vi "ColorGraphScale.vi"(11 "GraphRef":refnum<vi>) -> ()   [LabVIEW 2019]
uses:
  <vilib>/Utility/config.llb/Write Key (String).vi
  <vilib>/Utility/config.llb/Read Key (String).vi
  <vilib>/Utility/config.llb/NI_LVConfig.lvlib
panel:
  in  "Available Scales":u16(ring)
  in  "Load":bool
  in  "Scale Name":string
  in  "Save":bool
  in  "Add Aft":bool
  in  "SetMarker":bool
  in  "Rem":bool
  in  "Add Bef":bool
  in  "Max":dbl
  in  "Min":dbl
  in  "Marker Index":u16(ring) items=["1", "2", "3", "4", "5"]
  in  "TestData":dbl[][](array[numeric])
  in  "Test Data":bool
  in  "Quit":bool
  in  "InitProg":bool
  in  "Color":u32(colorbox)
  in  "ColorVal":u32 caption="Color Value"
  in  "MarkVal":dbl caption="Marker Value"
  out "error out":errorcluster caption="sortie d'erreur"
  in  "error in (no error)":errorcluster
  in  "Z.MarkVal":cluster{"MarkerVal":dbl, "ColorVal":u32}[](array[cluster])
  out "Graphe d'intensité":dbl[][](graph)
  # "ColorScale"
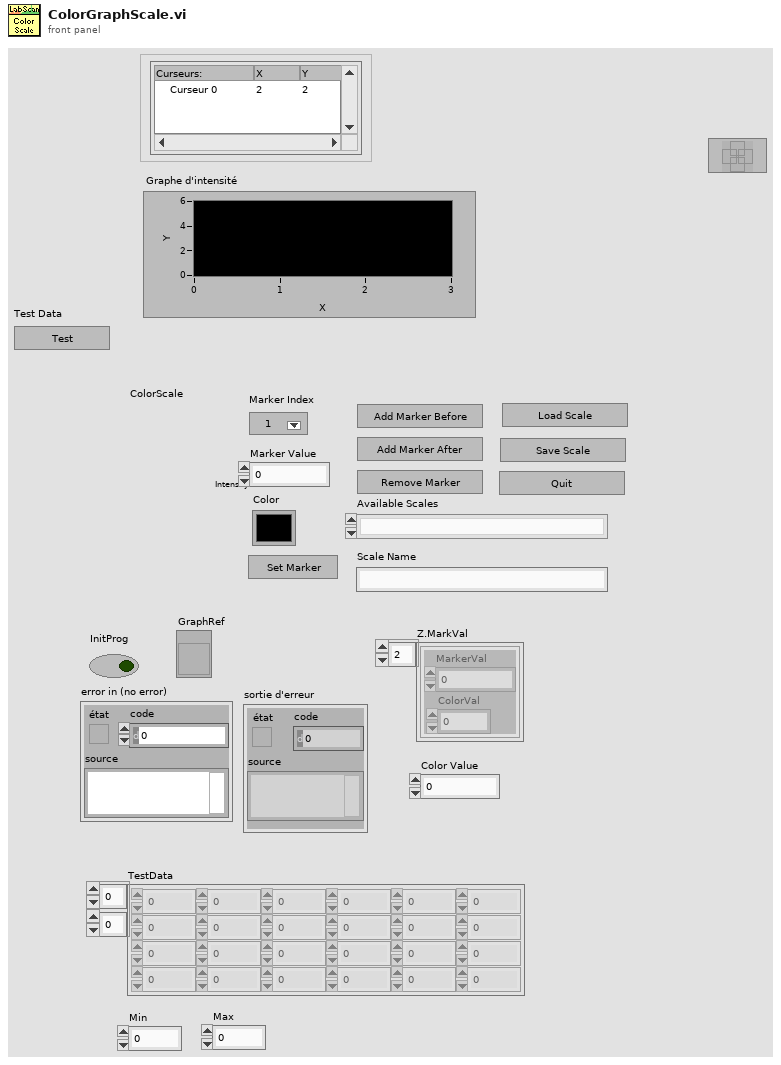
[diagram p1: front panel]
types:
  T1 = enum16{"Répertoire du VI actuel", "Répertoire du parent 1", "Répertoire du parent 2", "Répertoire du parent 3"}
  T2 = typedef "NI_LVConfig.lvlib/Config Data RefNum.ctl" = refnum<k1>
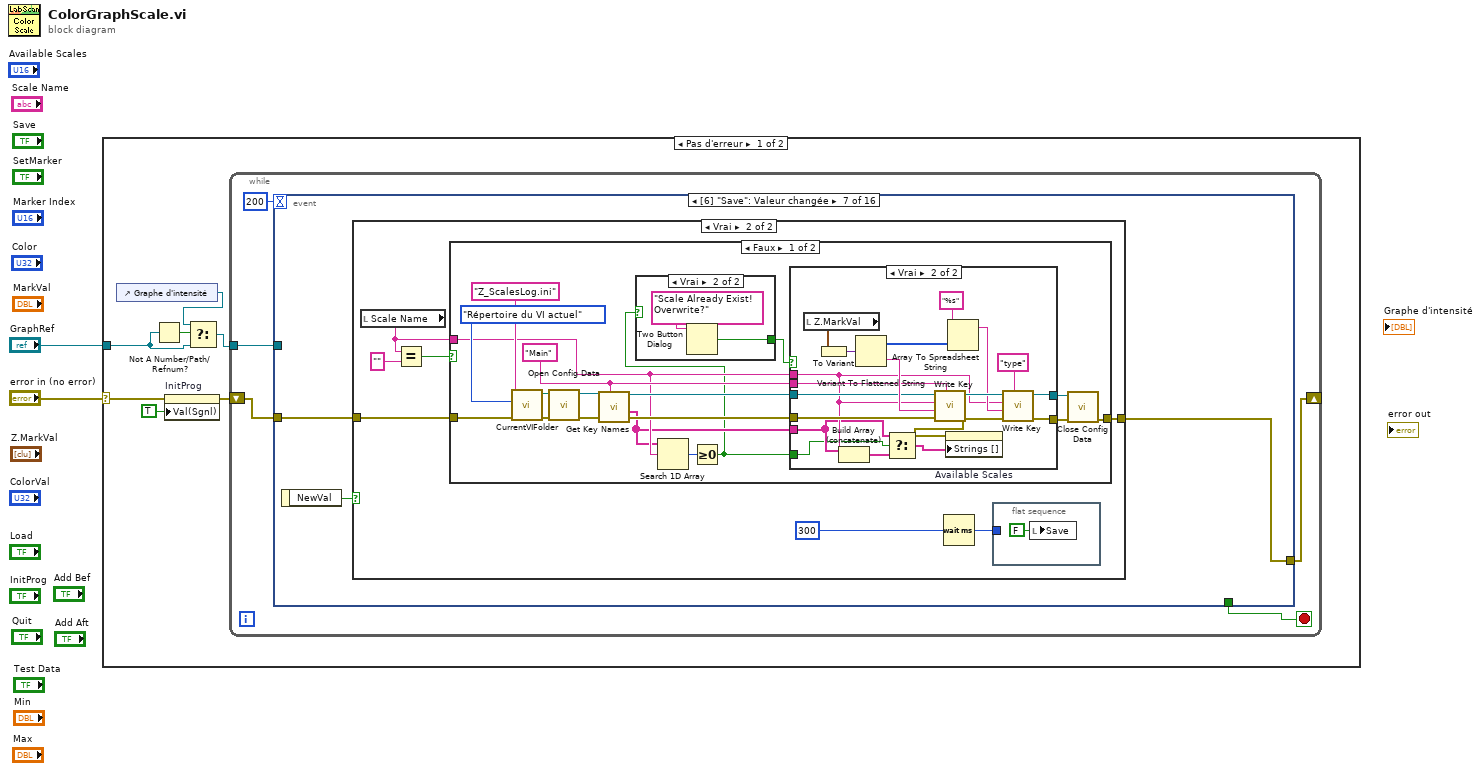
[diagram p0: block diagram]
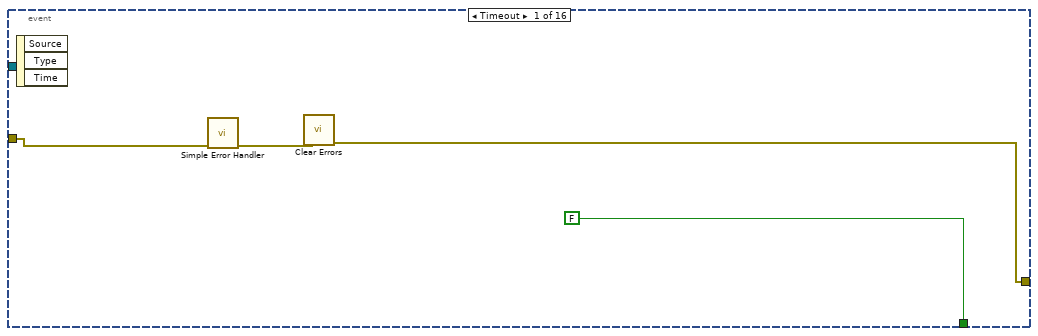
[diagram p2: hidden frame]
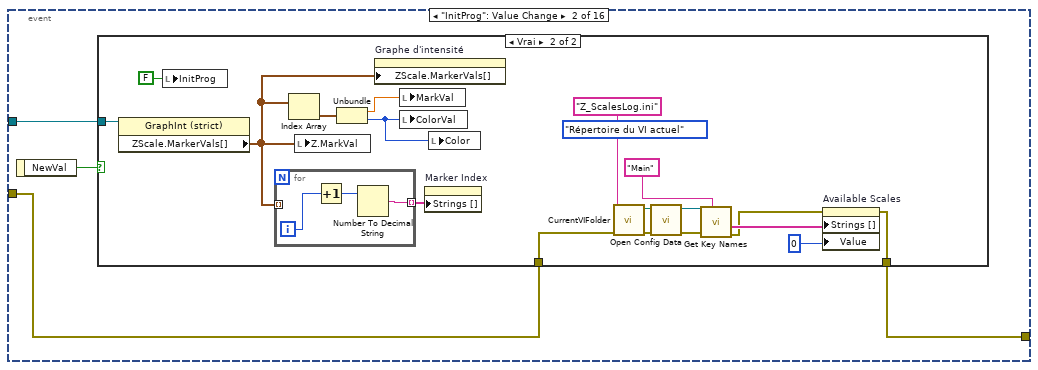
[diagram p3: hidden frame]
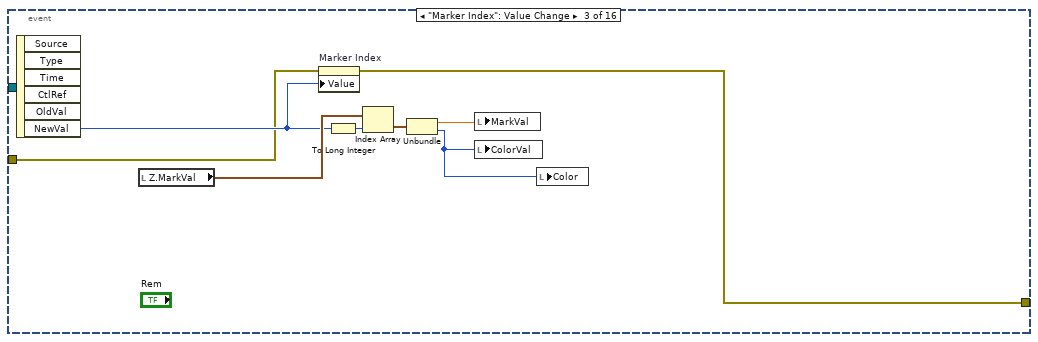
[diagram p5: hidden frame]
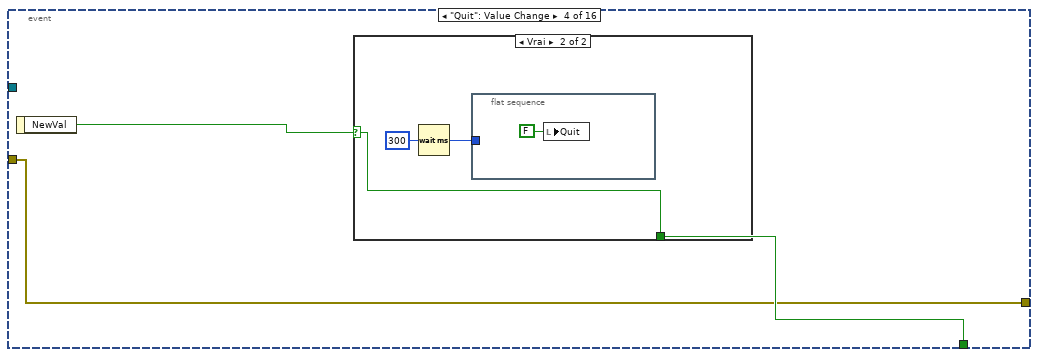
[diagram p6: hidden frame]
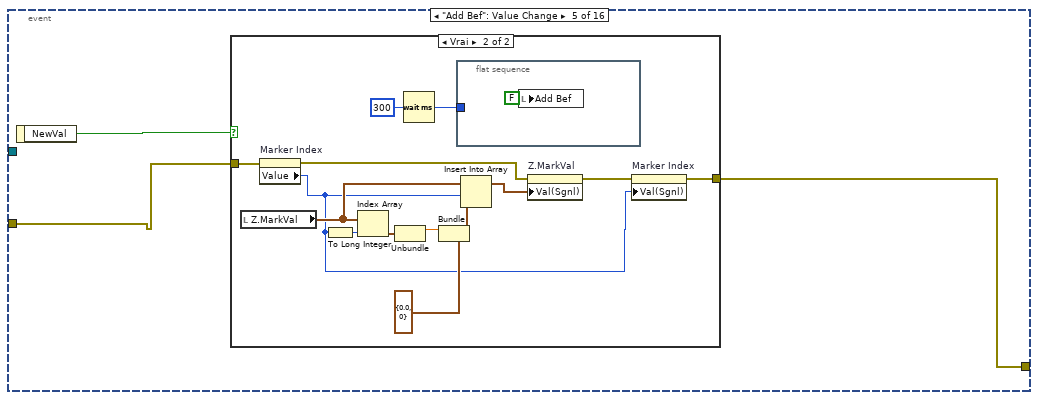
[diagram p8: hidden frame]
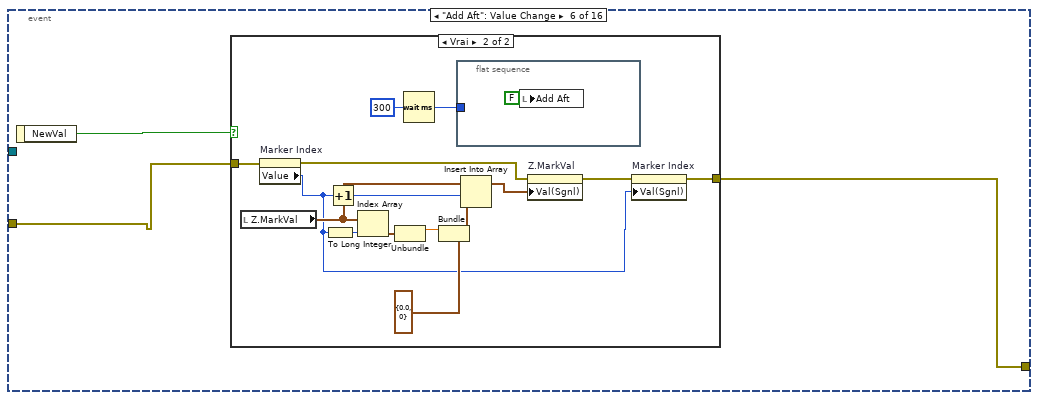
[diagram p10: hidden frame]
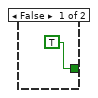
[diagram p13: hidden frame]
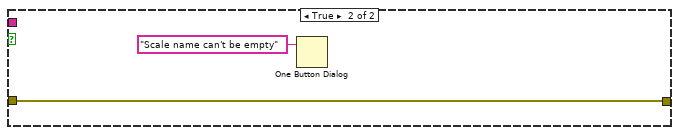
[diagram p15: hidden frame]
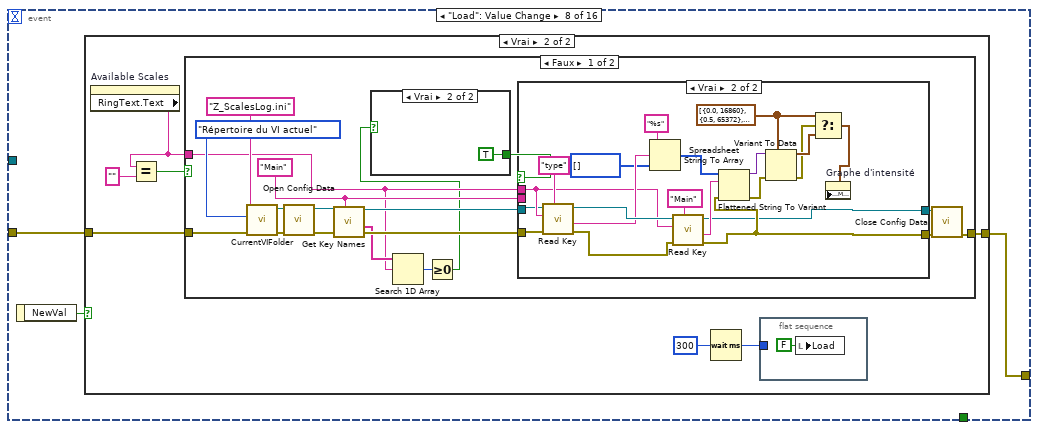
[diagram p16: hidden frame]
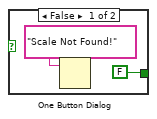
[diagram p18: hidden frame]
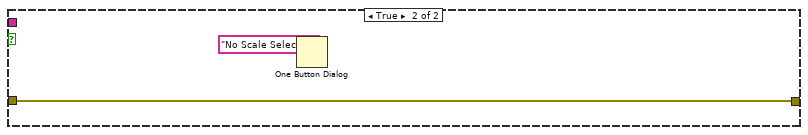
[diagram p20: hidden frame]
diagram:
  n1 = case shown="Pas d'erreur" "error in (no error)" {
    selector: "error in (no error)" -> [w9 _]
    tunnel: "GraphRef" -> [w5 _]
    frame No Error {
      n2 = control-ref of="Graphe d'intensité"() -> (w4:refnum<vi>)
      n3 = Not A Number/Path/Refnum?(number/path/refnum=w5) -> (NaN/Path/Refnum?=w6:bool)
      n4 = property on="InitProg" class="Bool (strict)"(error in=w9, "Val(Sgnl)"=TRUE ("Valeur (Signalisation)")) -> (error out=w8:errorcluster)  [unwired: 1 in, 1 out]
      n5 = Select(t=w4, s=w6, f=w5) -> (s? t:f=w3:refnum<vi>)
      n6 = while {
        shift-right: [w12] -> _
        shift-left: w8 -> [w11]
        tunnel: w3 -> [w10]
        stop <- w13 stop-if-true
        n7 = event shown="[6] \"Save\": Valeur changée" {
          selector: _ -> [_ _ _ _ _ _ _ _ _ _ _ _ _ _ _ _]
          dyn-events: _ -> [_ _ _ _ _ _ _ _ _ _ _ _ _ _ _ _]
          timeout: 200 -> [_ _ _ _ _ _ _ _ _ _ _ _ _ _ _ _]
          tunnel: [FALSE _ _ w54 _ _ _ _ _ _ _ _ _ _ _ _] -> w13
          tunnel: [w15 w20 w45 w53 w62 w81 w101 w157 w213 _ _ _ w243 w264 _ _] -> w12
          tunnel: w11 -> [w17 w19 w46 w53 w61 w80 w100 w156 w214 _ _ _ w247 w259 _ _]
          tunnel: w10 -> [_ w21 _ _ _ _ _ _ _ _ _ _ _ w263 _ _]
          event Timeout {
            n8 = event-data() -> ()  [unwired: 1 in, 3 out]
            n9 = call <vilib>:"Simple Error Handler.vi"("error in (no error)"=w17) -> ("error out"=w16:errorcluster)  [unwired: 4 in, 4 out]
            n10 = call <vilib>:"Clear Errors.vi"("error in (no error)"=w16) -> ("error out"=w15:errorcluster)  [unwired: 5 in, 1 out]
          }
          event "InitProg": Value Change {
            n11 = event-data() -> ("NewVal"=w22:bool)  [unwired: 1 in]
            n12 = case shown="Vrai" w22 {
              tunnel: w21 -> [_ w40]
              tunnel: w19 -> [w23 w26]
              tunnel: [w23 w25] -> w20
              frame False {
              }
              frame True {
                (unwired) T1."Répertoire du VI actuel" ("Source")
                n13 = property class="GraphInt (strict)"(reference=w40) -> ("ZScale.MarkerVals[]"=w35:cluster{dbl, u32}[])  [unwired: 1 in, 2 out]
                n14 = local write "InitProg"(FALSE ("InitProg")) -> ()
                n15 = for {
                  tunnel: [w43] -> w36 mode=indexing
                  tunnel: w35 -> [_] mode=indexing
                  i -> [w44]
                  n16 = Increment(x=w44) -> (x+1=w42:i32)
                  n17 = Number To Decimal String(number=w42) -> (decimal integer string=w43:string)  [unwired: 1 in]
                }
                n18 = Index Array(array=w35) -> (element=w39:cluster{dbl, u32})  [unwired: 1 in]
                n19 = local write "Z.MarkVal"(w35) -> ()
                n20 = Unbundle(w39) -> (w37:dbl, w38:u32)
                n21 = property on="Graphe d'intensité" class="GraphInt (strict)"("ZScale.MarkerVals[]"=w35) -> ()  [unwired: 2 in, 2 out]
                n22 = local write "MarkVal"(w37) -> ()
                n23 = local write "ColorVal"(w38) -> ()
                n24 = property on="Marker Index" class="MDér (strict)"("Strings []"=w36) -> ()  [unwired: 2 in, 2 out]
                n25 = local write "Color"(w38) -> ()
                n26 = call <userlib>:"CurrentVIFolder.vi"("error in (no error)"=w26, "NomFichier"="Z_ScalesLog.ini") -> ("error out"=w32:errorcluster, "Chemin"=w33:path)  [unwired: 7 in, 1 out]
                n27 = call <vilib>:"Open Config Data.vi"("error in (no error)"=w32, "configuration file path"=w33) -> ("error out"=w31:errorcluster, "refnum"=w30:T2)  [unwired: 7 in, 1 out]
                n28 = call <vilib>:"Get Key Names.vi"("section"="Main", "error in (no error)"=w31, "refnum"=w30) -> ("error out"=w27:errorcluster, "key names"=w28:string[])  [unwired: 5 in, 2 out]
                n29 = property on="Available Scales" class="MDér (strict)"(error in=w27, "Strings []"=w28, "Value"=0) -> (error out=w25:errorcluster)  [unwired: 1 in, 1 out]
              }
            }
          }
          event "Marker Index": Value Change {
            n30 = event-data() -> ("NewVal"=w47:u16)  [unwired: 1 in, 5 out]
            n31 = local read "Z.MarkVal"() -> (w52:cluster{"MarkerVal":dbl, "ColorVal":u32}[])
            n32 = property on="Marker Index" class="MDér (strict)"(error in=w46, "Value"=w47) -> (error out=w45:errorcluster)  [unwired: 1 in, 1 out]
            n33 = To Long Integer(number=w47) -> (32bit integer=w51:i32)
            n34 = Index Array(array=w52, index=w51) -> (element=w50:cluster{"MarkerVal":dbl, "ColorVal":u32})
            n35 = Unbundle(w50) -> ("MarkerVal"=w49:dbl, "ColorVal"=w48:u32)
            n36 = local write "MarkVal"(w49) -> ()
            n37 = local write "ColorVal"(w48) -> ()
            n38 = local write "Color"(w48) -> ()
          }
          event "Quit": Value Change {
            n39 = event-data() -> ("NewVal"=w55:bool)  [unwired: 1 in]
            n40 = case shown="Vrai" w55 {
              selector: w55 -> [w56 w59]
              tunnel: [w56 w59] -> w54
              frame False {
              }
              frame True {
                n41 = Wait (ms)(milliseconds to wait=u32 300 ("attente (ms)")) -> (millisecond timer value=w57:u32)
                n42 = flat-sequence {
                  tunnel: w57 -> [_]
                  frame #0 {
                    n43 = local write "Quit"(FALSE ("Quit")) -> ()
                  }
                }
              }
            }
          }
          event "Add Bef": Value Change {
            n44 = event-data() -> ("NewVal"=w63:bool)  [unwired: 1 in]
            n45 = case shown="Vrai" w63 {
              tunnel: w61 -> [w64 w73]
              tunnel: [w64 w74] -> w62
              frame False {
              }
              frame True {
                n46 = local read "Z.MarkVal"() -> (w70:cluster{"MarkerVal":dbl, "ColorVal":u32}[])
                n47 = property on="Marker Index" class="MDér (strict)"(error in=w73) -> (error out=w72:errorcluster, "Value"=w66:u16)  [unwired: 1 in, 1 out]
                n48 = To Long Integer(number=w66) -> (32bit integer=w65:i32)
                n49 = Index Array(array=w70, index=w65) -> (element=w69:cluster{"MarkerVal":dbl, "ColorVal":u32})
                n50 = Unbundle(w69) -> ("MarkerVal"=w67:dbl)  [unwired: 1 out]
                n51 = Wait (ms)(milliseconds to wait=u32 300 ("attente (ms)")) -> (millisecond timer value=w77:u32)
                n52 = Bundle(cluster=cluster{"MarkerVal":dbl, "ColorVal":u32} {"MarkerVal"=0.0, "ColorVal"=0}, "MarkerVal"=w67) -> (w68:cluster{"MarkerVal":dbl, "ColorVal":u32})  [unwired: 1 in]
                n53 = flat-sequence {
                  tunnel: w77 -> [_]
                  frame #0 {
                    n54 = local write "Add Bef"(FALSE ("Quit")) -> ()
                  }
                }
                n55 = Insert Into Array(array=w70, index=w66, new element=w68) -> (w75:cluster{"MarkerVal":dbl, "ColorVal":u32}[])
                n56 = property on="Z.MarkVal" class="Tabl (strict)"(error in=w72, "Val(Sgnl)"=w75) -> (error out=w76:errorcluster)  [unwired: 1 in, 1 out]
                n57 = property on="Marker Index" class="MDér (strict)"(error in=w76, "Val(Sgnl)"=w66) -> (error out=w74:errorcluster)  [unwired: 1 in, 1 out]
              }
            }
          }
          event "Add Aft": Value Change {
            n58 = event-data() -> ("NewVal"=w82:bool)  [unwired: 1 in]
            n59 = case shown="Vrai" w82 {
              tunnel: w80 -> [w83 w93]
              tunnel: [w83 w94] -> w81
              frame False {
              }
              frame True {
                n60 = local read "Z.MarkVal"() -> (w90:cluster{"MarkerVal":dbl, "ColorVal":u32}[])
                n61 = property on="Marker Index" class="MDér (strict)"(error in=w93) -> (error out=w92:errorcluster, "Value"=w84:u16)  [unwired: 1 in, 1 out]
                n62 = To Long Integer(number=w84) -> (32bit integer=w86:i32)
                n63 = Increment(x=w84) -> (x+1=w85:u16)
                n64 = Index Array(array=w90, index=w86) -> (element=w89:cluster{"MarkerVal":dbl, "ColorVal":u32})
                n65 = Unbundle(w89) -> ("MarkerVal"=w87:dbl)  [unwired: 1 out]
                n66 = Wait (ms)(milliseconds to wait=u32 300 ("attente (ms)")) -> (millisecond timer value=w97:u32)
                n67 = Bundle(cluster=cluster{"MarkerVal":dbl, "ColorVal":u32} {"MarkerVal"=0.0, "ColorVal"=0}, "MarkerVal"=w87) -> (w88:cluster{"MarkerVal":dbl, "ColorVal":u32})  [unwired: 1 in]
                n68 = flat-sequence {
                  tunnel: w97 -> [_]
                  frame #0 {
                    n69 = local write "Add Aft"(FALSE ("Quit")) -> ()
                  }
                }
                n70 = Insert Into Array(array=w90, index=w85, new element=w88) -> (w95:cluster{"MarkerVal":dbl, "ColorVal":u32}[])
                n71 = property on="Z.MarkVal" class="Tabl (strict)"(error in=w92, "Val(Sgnl)"=w95) -> (error out=w96:errorcluster)  [unwired: 1 in, 1 out]
                n72 = property on="Marker Index" class="MDér (strict)"(error in=w96, "Val(Sgnl)"=w84) -> (error out=w94:errorcluster)  [unwired: 1 in, 1 out]
              }
            }
          }
          event "Save": Value Change {
            n73 = event-data() -> ("NewVal"=w102:bool)  [unwired: 1 in]
            n74 = case shown="Vrai" w102 {
              tunnel: [w103 w109] -> w101
              tunnel: w100 -> [w103 w110]
              frame False {
              }
              frame True {
                n75 = local read "Scale Name"() -> (w104:string)
                n76 = Equal?(x=w104, y="") -> (x = y?=w105:bool)
                n77 = case shown="Faux" w105 {
                  tunnel: w110 -> [w126 w153]
                  tunnel: [w114 w153] -> w109
                  tunnel: w104 -> [w118 _]
                  frame False {
                    w119 = "Main" ("section")
                    n78 = call <userlib>:"CurrentVIFolder.vi"("error in (no error)"=w126, "Source"=T1."Répertoire du VI actuel", "NomFichier"="Z_ScalesLog.ini") -> ("error out"=w124:errorcluster, "Chemin"=w125:path)  [unwired: 6 in, 1 out]
                    n79 = call <vilib>:"Open Config Data.vi"("error in (no error)"=w124, "configuration file path"=w125) -> ("error out"=w123:errorcluster, "refnum"=w122:T2)  [unwired: 7 in, 1 out]
                    n80 = call <vilib>:"Get Key Names.vi"("section"=w119, "error in (no error)"=w123, "refnum"=w122) -> ("error out"=w121:errorcluster, "key names"=w112:string[], "refnum out"=w120:T2)  [unwired: 5 in, 1 out]
                    n81 = Search 1D Array(1D array=w112, element=w118) -> (index of element=w117:i32)  [unwired: 1 in]
                    n82 = Greater Or Equal To 0?(x=w117) -> (x >= 0?=w111:bool)
                    n83 = case shown="Vrai" w111 {
                      tunnel: [TRUE ("T button?") w130] -> w113
                      frame False {
                      }
                      frame True {
                        n84 = Two Button Dialog(message="Scale Already Exist! Overwrite?") -> (T button?=w130:bool)  [unwired: 2 in]
                      }
                    }
                    n85 = case shown="Vrai" w113 {
                      tunnel: w121 -> [w132 w144]
                      tunnel: w120 -> [w133 w143]
                      tunnel: w119 -> [_ w142]
                      tunnel: w118 -> [_ w138]
                      tunnel: [w132 w141] -> w116
                      tunnel: [w133 w140] -> w115
                      tunnel: w112 -> [_ w136]
                      tunnel: w111 -> [_ w135]
                      frame False {
                      }
                      frame True {
                        n86 = local read "Z.MarkVal"() -> (w152:cluster{"MarkerVal":dbl, "ColorVal":u32}[])
                        n87 = To Variant(anything=w152) -> (Variant=w151:variant)
                        n88 = Build Array (concatenate)(w136, w138) -> (w137:string[])
                        n89 = Variant To Flattened String(Variant=w151) -> (data string=w150:string, 1:w147:i16[])
                        n90 = Select(t=w136, s=w135, f=w137) -> (s? t:f=w134:string[])
                        n91 = call-poly <vilib>:"Write Key.vi"("section"=w142, "error in (no error)"=w144, "value"=w150, "key"=w138, "refnum"=w143) -> ("error out"=w139:errorcluster, "refnum out"=w148:T2)  [unwired: 4 in, 1 out]
                        n92 = property on="Available Scales" class="MDér (strict)"(error in=w139, "Strings []"=w134) -> ()  [unwired: 1 in, 2 out]
                        n93 = Array To Spreadsheet String(array=w147, 3:"%s" ("chaîne de format")) -> (spreadsheet string=w146:string)  [unwired: 1 in]
                        n94 = call-poly <vilib>:"Write Key.vi"("section"="type", "error in (no error)"=w139, "value"=w146, "key"=w138, "refnum"=w148) -> ("error out"=w141:errorcluster, "refnum out"=w140:T2)  [unwired: 4 in, 1 out]
                      }
                    }
                    n95 = call <vilib>:"Close Config Data.vi"("error in (no error)"=w116, "refnum"=w115) -> ("error out"=w114:errorcluster)  [unwired: 8 in, 1 out]
                  }
                  frame True {
                    n96 = One Button Dialog(message="Scale name can't be empty") -> ()  [unwired: 1 in, 1 out]
                  }
                }
                n97 = Wait (ms)(milliseconds to wait=u32 300 ("attente (ms)")) -> (millisecond timer value=w108:u32)
                n98 = flat-sequence {
                  tunnel: w108 -> [_]
                  frame #0 {
                    n99 = local write "Save"(FALSE ("Save")) -> ()
                  }
                }
              }
            }
          }
          event "Load": Value Change {
            n100 = event-data() -> ("NewVal"=w158:bool)  [unwired: 1 in]
            n101 = case shown="Vrai" w158 {
              tunnel: [w159 w165] -> w157
              tunnel: w156 -> [w159 w166]
              frame False {
              }
              frame True {
                n102 = property on="Available Scales" class="MDér (strict)"() -> ("RingText.Text"=w160:string)  [unwired: 2 in, 2 out]
                n103 = Equal?(x=w160, y="") -> (x = y?=w161:bool)
                n104 = case shown="Faux" w161 {
                  tunnel: w166 -> [w182 w210]
                  tunnel: [w169 w210] -> w165
                  tunnel: w160 -> [w173 _]
                  frame False {
                    w174 = "Main" ("section")
                    n105 = call <userlib>:"CurrentVIFolder.vi"("error in (no error)"=w182, "Source"=T1."Répertoire du VI actuel", "NomFichier"="Z_ScalesLog.ini") -> ("error out"=w180:errorcluster, "Chemin"=w181:path)  [unwired: 6 in, 1 out]
                    n106 = call <vilib>:"Open Config Data.vi"("error in (no error)"=w180, "configuration file path"=w181) -> ("error out"=w179:errorcluster, "refnum"=w178:T2)  [unwired: 7 in, 1 out]
                    n107 = call <vilib>:"Get Key Names.vi"("section"=w174, "error in (no error)"=w179, "refnum"=w178) -> ("error out"=w177:errorcluster, "key names"=w175:string[], "refnum out"=w176:T2)  [unwired: 5 in, 1 out]
                    n108 = Search 1D Array(1D array=w175, element=w173) -> (index of element=w172:i32)  [unwired: 1 in]
                    n109 = Greater Or Equal To 0?(x=w172) -> (x >= 0?=w168:bool)
                    n110 = case shown="Vrai" w168 {
                      tunnel: [FALSE TRUE ("T button?")] -> w167
                      frame False {
                        n111 = One Button Dialog(message="Scale Not Found!") -> ()  [unwired: 1 in, 1 out]
                      }
                      frame True {
                      }
                    }
                    n112 = case shown="Vrai" w167 {
                      tunnel: w177 -> [w188 w195]
                      tunnel: w176 -> [w189 w190]
                      tunnel: w174 -> [_ _]
                      tunnel: w173 -> [_ w193]
                      tunnel: [w188 w194] -> w171
                      tunnel: [w189 w192] -> w170
                      frame False {
                      }
                      frame True {
                        w198 = cluster{"MarkerVal":dbl, "ColorVal":u32}[] [{"MarkerVal"=0.0, "ColorVal"=16860}, {"MarkerVal"=0.5, "ColorVal"=65372}, {"MarkerVal"=1.0, "ColorVal"=16776793}] ("Z.MarkVal")
                        n113 = call-poly <vilib>:"Read Key.vi"("section"="type", "error in (no error)"=w195, "key"=w193, "refnum"=w190) -> ("error out"=w204:errorcluster, "value"=w205:string, "refnum out"=w206:T2)  [unwired: 4 in, 1 out]
                        n114 = Spreadsheet String To Array(format string="%s" ("chaîne de format"), spreadsheet string=w205, array type (2D Dbl)=i16[] [] ("chaîne de type")) -> (array=w202:i16[])  [unwired: 1 in]
                        n115 = call-poly <vilib>:"Read Key.vi"("section"="Main", "error in (no error)"=w204, "key"=w193, "refnum"=w206) -> ("error out"=w194:errorcluster, "value"=w208:string, "refnum out"=w192:T2)  [unwired: 4 in, 1 out]
                        n116 = Flattened String To Variant(4:w194, 6:w208, 7:w202) -> (0:w200:errorcluster, 3:w201:variant)
                        n117 = Variant To Data(error in=w200, type=w198, Variant=w201) -> (data=w197:cluster{"MarkerVal":dbl, "ColorVal":u32}[], error out=w196:errorcluster)
                        n118 = Select(t=w198, s=w196, f=w197) -> (s? t:f=w191:cluster{"MarkerVal":dbl, "ColorVal":u32}[])
                        n119 = property on="Graphe d'intensité" class="GraphInt (strict)"("ZScale.MarkerVals[]"=w191) -> ()  [unwired: 2 in, 2 out]
                      }
                    }
                    n120 = call <vilib>:"Close Config Data.vi"("error in (no error)"=w171, "refnum"=w170) -> ("error out"=w169:errorcluster)  [unwired: 8 in, 1 out]
                  }
                  frame True {
                    n121 = One Button Dialog(message="No Scale Selected") -> ()  [unwired: 1 in, 1 out]
                  }
                }
                n122 = Wait (ms)(milliseconds to wait=u32 300 ("attente (ms)")) -> (millisecond timer value=w164:u32)
                n123 = flat-sequence {
                  tunnel: w164 -> [_]
                  frame #0 {
                    n124 = local write "Load"(FALSE ("Save")) -> ()
                  }
                }
              }
            }
          }
          event "Rem": Value Change {
            n125 = event-data() -> ("NewVal"=w215:bool)  [unwired: 1 in]
            n126 = case shown="Vrai" w215 {
              tunnel: w214 -> [w216 w225]
              tunnel: [w216 w224] -> w213
              frame False {
              }
              frame True {
                n127 = property on="Marker Index" class="MDér (strict)"() -> ("Value"=w218:u16)  [unwired: 2 in, 2 out]
                n128 = local read "Z.MarkVal"() -> (w223:cluster{"MarkerVal":dbl, "ColorVal":u32}[])
                n129 = Wait (ms)(milliseconds to wait=u32 300 ("attente (ms)")) -> (millisecond timer value=w227:u32)
                n130 = Greater Than 0?(x=w218) -> (x > 0?=w219:bool)
                n131 = Delete From Array(array=w223, length=1 ("longueur"), index=w218) -> (array with subset deleted=w222:cluster{"MarkerVal":dbl, "ColorVal":u32}[])  [unwired: 1 out]
                n132 = flat-sequence {
                  tunnel: w227 -> [_]
                  frame #0 {
                    n133 = local write "Rem"(FALSE ("Quit")) -> ()
                  }
                }
                n134 = Decrement(x=w218) -> (x-1=w220:u16)
                n135 = Select(t=w220, s=w219, f=w218) -> (s? t:f=w217:u16)
                n136 = property on="Z.MarkVal" class="Tabl (strict)"(error in=w225, "Val(Sgnl)"=w222) -> (error out=w226:errorcluster)  [unwired: 1 in, 1 out]
                n137 = property on="Marker Index" class="MDér (strict)"(error in=w226, "Val(Sgnl)"=w217) -> (error out=w224:errorcluster)  [unwired: 1 in, 1 out]
              }
            }
          }
          event "SetMarker": Value Change {
            n138 = event-data() -> ("NewVal"=w230:bool)  [unwired: 1 in, 5 out]
            n139 = case shown="Vrai" w230 {
              frame False {
              }
              frame True {
                n140 = local read "Z.MarkVal"() -> (w234:cluster{"MarkerVal":dbl, "ColorVal":u32}[])
                n141 = local read "Marker Index"() -> (w233:u16)
                n142 = local read "ColorVal"() -> (w235:u32)
                n143 = local read "MarkVal"() -> (w236:dbl)
                n144 = Wait (ms)(milliseconds to wait=u32 300 ("attente (ms)")) -> (millisecond timer value=w237:u32)
                n145 = flat-sequence {
                  tunnel: w237 -> [_]
                  frame #0 {
                    n146 = local write "SetMarker"(FALSE ("Quit")) -> ()
                  }
                }
                n147 = Bundle("MarkVal"=w236, "ColorVal"=w235) -> (w232:cluster{"MarkVal":dbl, "ColorVal":u32})  [unwired: 1 in]
                n148 = Replace Array Subset(array=w234, new element=w232, index=w233) -> (w231:cluster{"MarkerVal":dbl, "ColorVal":u32}[])
                n149 = property on="Z.MarkVal" class="Tabl (strict)"("Val(Sgnl)"=w231) -> ()  [unwired: 2 in, 2 out]
              }
            }
          }
          event "Color": Value Change {
            n150 = event-data() -> ("NewVal"=w240:u32)  [unwired: 1 in, 5 out]
            n151 = local write "ColorVal"(w240) -> ()
          }
          event "ColorVal": Value Change {
            n152 = event-data() -> ("NewVal"=w241:u32)  [unwired: 1 in, 5 out]
            n153 = local write "Color"(w241) -> ()
          }
          event "Test Data": Value Change {
            n154 = event-data() -> ("NewVal"=w250:bool)  [unwired: 1 in]
            n155 = case shown="Vrai" w250 {
              tunnel: [w251 w253] -> w248
              tunnel: w247 -> [w251 w253]
              tunnel: "TestData" -> [_ w252]
              frame False {
              }
              frame True {
                n156 = local write "Graphe d'intensité"(w252) -> ()
                n157 = Wait (ms)(milliseconds to wait=u32 300 ("attente (ms)")) -> (millisecond timer value=w255:u32)
                n158 = flat-sequence {
                  tunnel: w255 -> [_]
                  frame #0 {
                    n159 = local write "Test Data"(FALSE ("Quit")) -> ()
                  }
                }
              }
            }
            n160 = property on="Graphe d'intensité" class="GraphInt (strict)"(error in=w248) -> (error out=w244:errorcluster, "ZScale.MarkerVals[]"=w249:cluster{dbl, u32}[])  [unwired: 1 in, 1 out]
            n161 = property on="Z.MarkVal" class="Tabl (strict)"(error in=w244, "Val(Sgnl)"=w249) -> (error out=w246:errorcluster)  [unwired: 1 in, 1 out]
            n162 = property on="Marker Index" class="MDér (strict)"(error in=w246, "Val(Sgnl)"=u16 0 ("Valeur (Signalisation)")) -> (error out=w243:errorcluster)  [unwired: 1 in, 1 out]
          }
          event "Z.MarkVal": Value Change {
            n163 = event-data() -> ("NewVal"=w262:cluster{"MarkerVal":dbl, "ColorVal":u32}[])  [unwired: 1 in]
            n164 = property on="Marker Index" class="MDér (strict)"(error in=w259) -> (error out=w258:errorcluster, "Value"=w257:u16)  [unwired: 1 in, 1 out]
            n165 = for {
              tunnel: [w267] -> w265 mode=indexing
              tunnel: w262 -> [_] mode=indexing
              i -> [w268]
              n166 = Increment(x=w268) -> (x+1=w266:i32)
              n167 = Number To Decimal String(number=w266) -> (decimal integer string=w267:string)  [unwired: 1 in]
            }
            n168 = property on="Nœud de propriété" class="GraphInt (strict)"(reference=w263, error in=w258, "ZScale.MarkerVals[]"=w262) -> (error out=w261:errorcluster)  [unwired: 1 out]
            n169 = property on="Graphe d'intensité" class="GraphInt (strict)"(error in=w261, "ZScale.MarkerVals[]"=w262) -> (error out=w260:errorcluster)  [unwired: 1 in, 1 out]
            n170 = property on="Marker Index" class="MDér (strict)"(error in=w260, "Strings []"=w265, "Value"=w257) -> (error out=w264:errorcluster)  [unwired: 1 in, 1 out]
          }
          event "Min": Value Change {
            n171 = event-data() -> ("NewVal"=w278:dbl)  [unwired: 1 in]
            n172 = local read "Max"() -> (w279:dbl)
            n173 = local read "TestData"() -> (w280:dbl[][])
            n174 = Array Size(array=w280) -> (size(s)=w272:i32[])
            n175 = Subtract(x=w279, y=w278) -> (x-y=w277:dbl)
            n176 = Multiply Array Elements(1:w272) -> (0:w276:i32)
            n177 = Divide(x=w277, y=w276) -> (x/y=w275:dbl)
            n178 = for {
              N: w276 -> [_]
              tunnel: w275 -> [w282]
              tunnel: [w281] -> w274 mode=indexing
              i -> [w283]
              n179 = Multiply(x=w282, y=w283) -> (x*y=w281:dbl)
            }
            n180 = Index Array(array=w272) -> (element #1=w271:i32, element #2=w270:i32)  [unwired: 2 in]
            n181 = Reshape Array(w274, w271, w270) -> (w273:dbl[][])
            n182 = property on="Test Data" class="Bool (strict)"("Val(Sgnl)"=TRUE ("Valeur (Signalisation)")) -> ()  [unwired: 2 in, 2 out]
            n183 = local write "TestData"(w273) -> ()
          }
          event "Max": Value Change {
            n184 = event-data() -> ("NewVal"=w285:dbl)  [unwired: 1 in]
            n185 = local read "Min"() -> (w284:dbl)
            n186 = local read "TestData"() -> (w295:dbl[][])
            n187 = Array Size(array=w295) -> (size(s)=w289:i32[])
            n188 = Subtract(x=w285, y=w284) -> (x-y=w294:dbl)
            n189 = Multiply Array Elements(1:w289) -> (0:w293:i32)
            n190 = Divide(x=w294, y=w293) -> (x/y=w292:dbl)
            n191 = for {
              N: w293 -> [_]
              tunnel: w292 -> [w297]
              tunnel: [w296] -> w291 mode=indexing
              i -> [w298]
              n192 = Multiply(x=w297, y=w298) -> (x*y=w296:dbl)
            }
            n193 = Index Array(array=w289) -> (element #1=w288:i32, element #2=w287:i32)  [unwired: 2 in]
            n194 = Reshape Array(w291, w288, w287) -> (w290:dbl[][])
            n195 = property on="Test Data" class="Bool (strict)"("Val(Sgnl)"=TRUE ("Valeur (Signalisation)")) -> ()  [unwired: 2 in, 2 out]
            n196 = local write "TestData"(w290) -> ()
          }
        }
      }
    }
    frame Error {
    }
  }
